vi "VI Server_SetCursorToBusy.vi"(8 "error in (no error)":errorcluster, 11 "VI Server Cluster":T1) -> (0 "error out":errorcluster, 3 "VI Server Cluster.DUP":T1)   [LabVIEW 2020, in "VI Server Toolkit LV2013.lvlib"]
doc: "Sets cursor to \"Busy\" from VI Server Cluster input."
uses:
  VI Server Toolkit LV2013.lvlib
  VI Server_TypeDefs/VI Server_RefsCluster.ctl
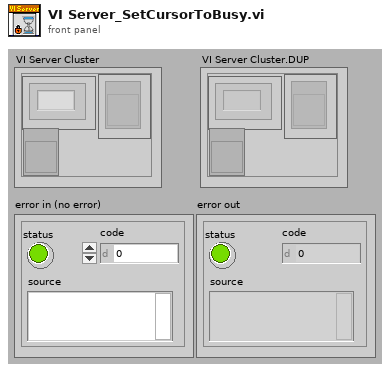
[diagram p1: front panel]
types:
  T1 = typedef "VI Server_RefsCluster.ctl" = cluster{"Labels":string[], "Refs":refnum<vi>[], "VI Ref":refnum<vi>}
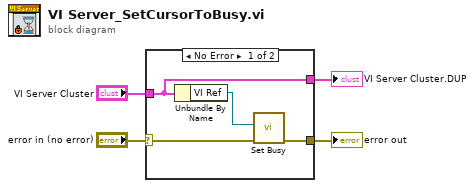
[diagram p0: block diagram]
diagram:
  n1 = case shown="No Error" "error in (no error)" {
    selector: "error in (no error)" -> [w5 w9]
    tunnel: [w8 w9] -> w4
    tunnel: "VI Server Cluster" -> [w6 _]
    tunnel: [w6 _] -> w2
    frame No Error {
      n2 = Unbundle By Name(w6) -> ("VI Ref"=w7:refnum<vi>)
      n3 = call <vilib>:"Set Busy.vi"("error in (no error)"=w5, "VI reference (current VI)"=w7) -> ("error out"=w8:errorcluster)  [unwired: 8 in, 1 out]
    }
    frame Error {
    }
  }
  "VI Server Cluster.DUP" <- w2
  "error out" <- w4
